vi "Icon_Calculate Height and Width.vi"(4 "Region":T1) -> (1 "Region Out":T1)   [LabVIEW 2009]
uses:
  Controls/Cluster/Cluster_Region info.ctl
  Controls/Cluster/Cluster_Top Left position.ctl
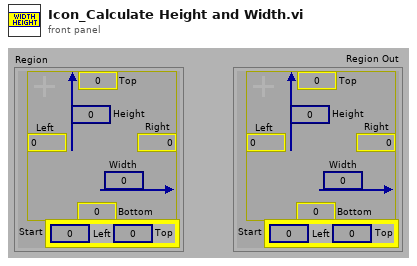
[diagram p1: front panel]
types:
  T1 = typedef "Cluster_Region info.ctl" = cluster{"Left":i32, "Top":i32, "Right":i32, "Bottom":i32, "Width":u32, "Height":u32, "Start":T2}
  T2 = typedef "Cluster_Top Left position.ctl" = cluster{"Left":i32, "Top":i32}
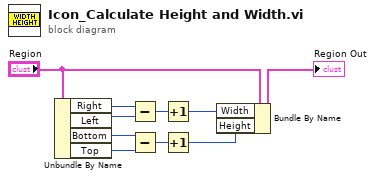
[diagram p0: block diagram]
diagram:
  n1 = Unbundle By Name("Region") -> ("Right"=w10:i32, "Left"=w9:i32, "Bottom"=w6:i32, "Top"=w5:i32)
  n2 = Subtract(x=w10, y=w9) -> (x-y=w7:i32)
  n3 = Subtract(x=w6, y=w5) -> (x-y=w8:i32)
  n4 = Increment(x=w7) -> (x+1=w3:i32)
  n5 = Increment(x=w8) -> (x+1=w4:i32)
  n6 = Bundle By Name(cluster="Region", "Width"=w3, "Height"=w4) -> (→"Region Out":T1)
